vi "Setup Cursors.vi"(8 "error in (no error)":errorcluster, 11 "data":waveform(dbl)[](array[waveform])) -> (0 "error out":errorcluster, 1 "Cursor List 2":T1(array[cluster]), 2 "Cursor List":T1(array[cluster]), 3 "waveform out":waveform(dbl), 5 "duration":dbl)   [LabVIEW 2020]
uses:
  <vilib>/Waveform/WDTOps.llb/WDT Waveform Duration DBL.vi
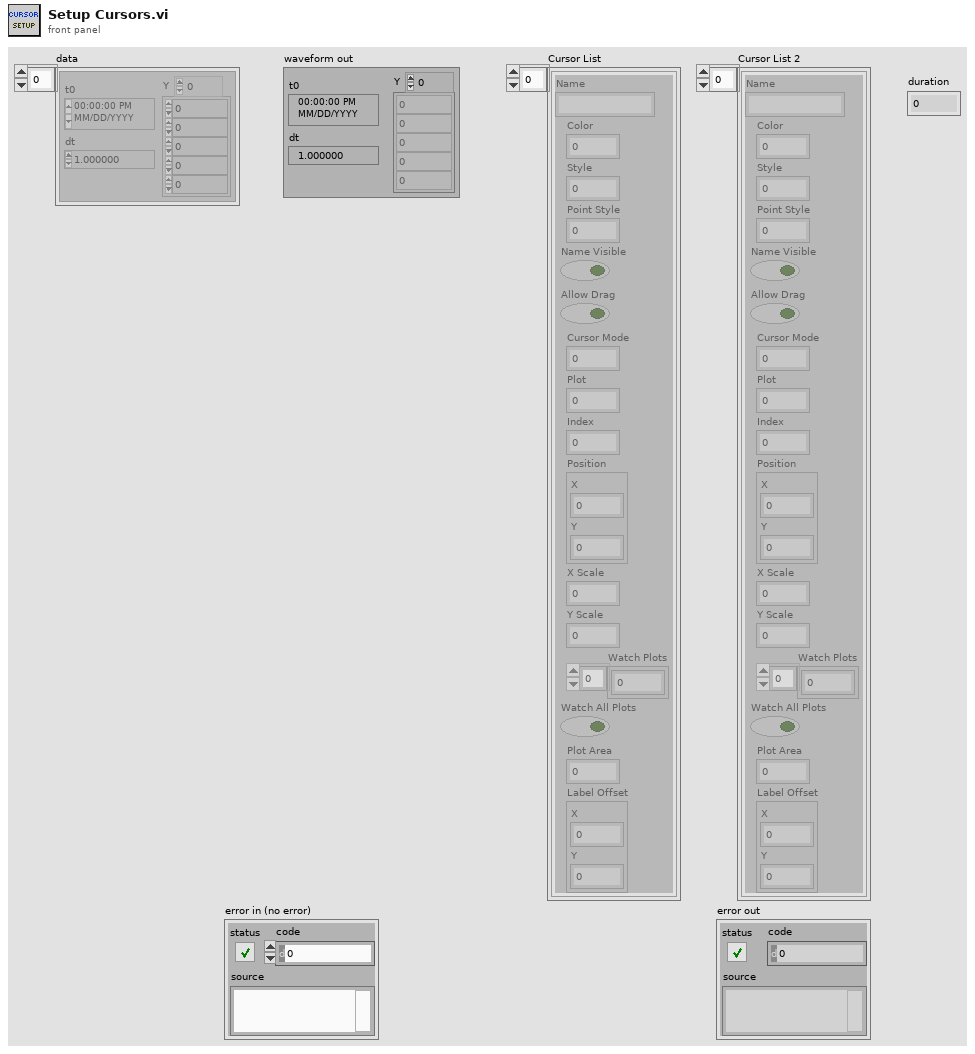
[diagram p1: front panel]
types:
  T1 = cluster{"Name":string, "Color":u32, "Style":u8, "Point Style":u8, "Name Visible":bool, "Allow Drag":bool, "Cursor Mode":u32, "Plot":i32, "Index":i32, "Position":cluster{"X":dbl, "Y":dbl}, "X Scale":u32, "Y Scale":u32, "Watch Plots":i32[], "Watch All Plots":bool, "Plot Area":i32, "Label Offset":cluster{"X":dbl, "Y":dbl}}[]
  T2 = cluster{"Name":string, "Color":u32, "Style":u8, "Point Style":u8, "Name Visible":bool, "Allow Drag":bool, "Cursor Mode":u32, "Plot":i32, "Index":i32, "Position":cluster{"X":dbl, "Y":dbl}, "X Scale":u32, "Y Scale":u32, "Watch Plots":i32[], "Watch All Plots":bool, "Plot Area":i32, "Label Offset":cluster{"X":dbl, "Y":dbl}}
  T3 = cluster{"Cursor List[0]":cluster{"Name":string, "Color":u32, "Style":u8, "Point Style":u8, "Name Visible":bool, "Allow Drag":bool, "Cursor Mode":u32, "Plot":i32, "Index":i32, "Position":cluster{"X":dbl, "Y":dbl}, "X Scale":u32, "Y Scale":u32, "Watch Plots":i32[], "Watch All Plots":bool, "Plot Area":i32, "Label Offset":cluster{"X":dbl, "Y":dbl}}, "Cursor List[1]":cluster{"Name":string, "Color":u32, "Style":u8, "Point Style":u8, "Name Visible":bool, "Allow Drag":bool, "Cursor Mode":u32, "Plot":i32, "Index":i32, "Position":cluster{"X":dbl, "Y":dbl}, "X Scale":u32, "Y Scale":u32, "Watch Plots":i32[], "Watch All Plots":bool, "Plot Area":i32, "Label Offset":cluster{"X":dbl, "Y":dbl}}, "Cursor List[2]":cluster{"Name":string, "Color":u32, "Style":u8, "Point Style":u8, "Name Visible":bool, "Allow Drag":bool, "Cursor Mode":u32, "Plot":i32, "Index":i32, "Position":cluster{"X":dbl, "Y":dbl}, "X Scale":u32, "Y Scale":u32, "Watch Plots":i32[], "Watch All Plots":bool, "Plot Area":i32, "Label Offset":cluster{"X":dbl, "Y":dbl}}, "Cursor List[3]":cluster{"Name":string, "Color":u32, "Style":u8, "Point Style":u8, "Name Visible":bool, "Allow Drag":bool, "Cursor Mode":u32, "Plot":i32, "Index":i32, "Position":cluster{"X":dbl, "Y":dbl}, "X Scale":u32, "Y Scale":u32, "Watch Plots":i32[], "Watch All Plots":bool, "Plot Area":i32, "Label Offset":cluster{"X":dbl, "Y":dbl}}, "Cursor List[4]":cluster{"Name":string, "Color":u32, "Style":u8, "Point Style":u8, "Name Visible":bool, "Allow Drag":bool, "Cursor Mode":u32, "Plot":i32, "Index":i32, "Position":cluster{"X":dbl, "Y":dbl}, "X Scale":u32, "Y Scale":u32, "Watch Plots":i32[], "Watch All Plots":bool, "Plot Area":i32, "Label Offset":cluster{"X":dbl, "Y":dbl}}, "Cursor List[5]":cluster{"Name":string, "Color":u32, "Style":u8, "Point Style":u8, "Name Visible":bool, "Allow Drag":bool, "Cursor Mode":u32, "Plot":i32, "Index":i32, "Position":cluster{"X":dbl, "Y":dbl}, "X Scale":u32, "Y Scale":u32, "Watch Plots":i32[], "Watch All Plots":bool, "Plot Area":i32, "Label Offset":cluster{"X":dbl, "Y":dbl}}, "Cursor List[6]":cluster{"Name":string, "Color":u32, "Style":u8, "Point Style":u8, "Name Visible":bool, "Allow Drag":bool, "Cursor Mode":u32, "Plot":i32, "Index":i32, "Position":cluster{"X":dbl, "Y":dbl}, "X Scale":u32, "Y Scale":u32, "Watch Plots":i32[], "Watch All Plots":bool, "Plot Area":i32, "Label Offset":cluster{"X":dbl, "Y":dbl}}, "Cursor List[7]":cluster{"Name":string, "Color":u32, "Style":u8, "Point Style":u8, "Name Visible":bool, "Allow Drag":bool, "Cursor Mode":u32, "Plot":i32, "Index":i32, "Position":cluster{"X":dbl, "Y":dbl}, "X Scale":u32, "Y Scale":u32, "Watch Plots":i32[], "Watch All Plots":bool, "Plot Area":i32, "Label Offset":cluster{"X":dbl, "Y":dbl}}, "Cursor List[8]":cluster{"Name":string, "Color":u32, "Style":u8, "Point Style":u8, "Name Visible":bool, "Allow Drag":bool, "Cursor Mode":u32, "Plot":i32, "Index":i32, "Position":cluster{"X":dbl, "Y":dbl}, "X Scale":u32, "Y Scale":u32, "Watch Plots":i32[], "Watch All Plots":bool, "Plot Area":i32, "Label Offset":cluster{"X":dbl, "Y":dbl}}}
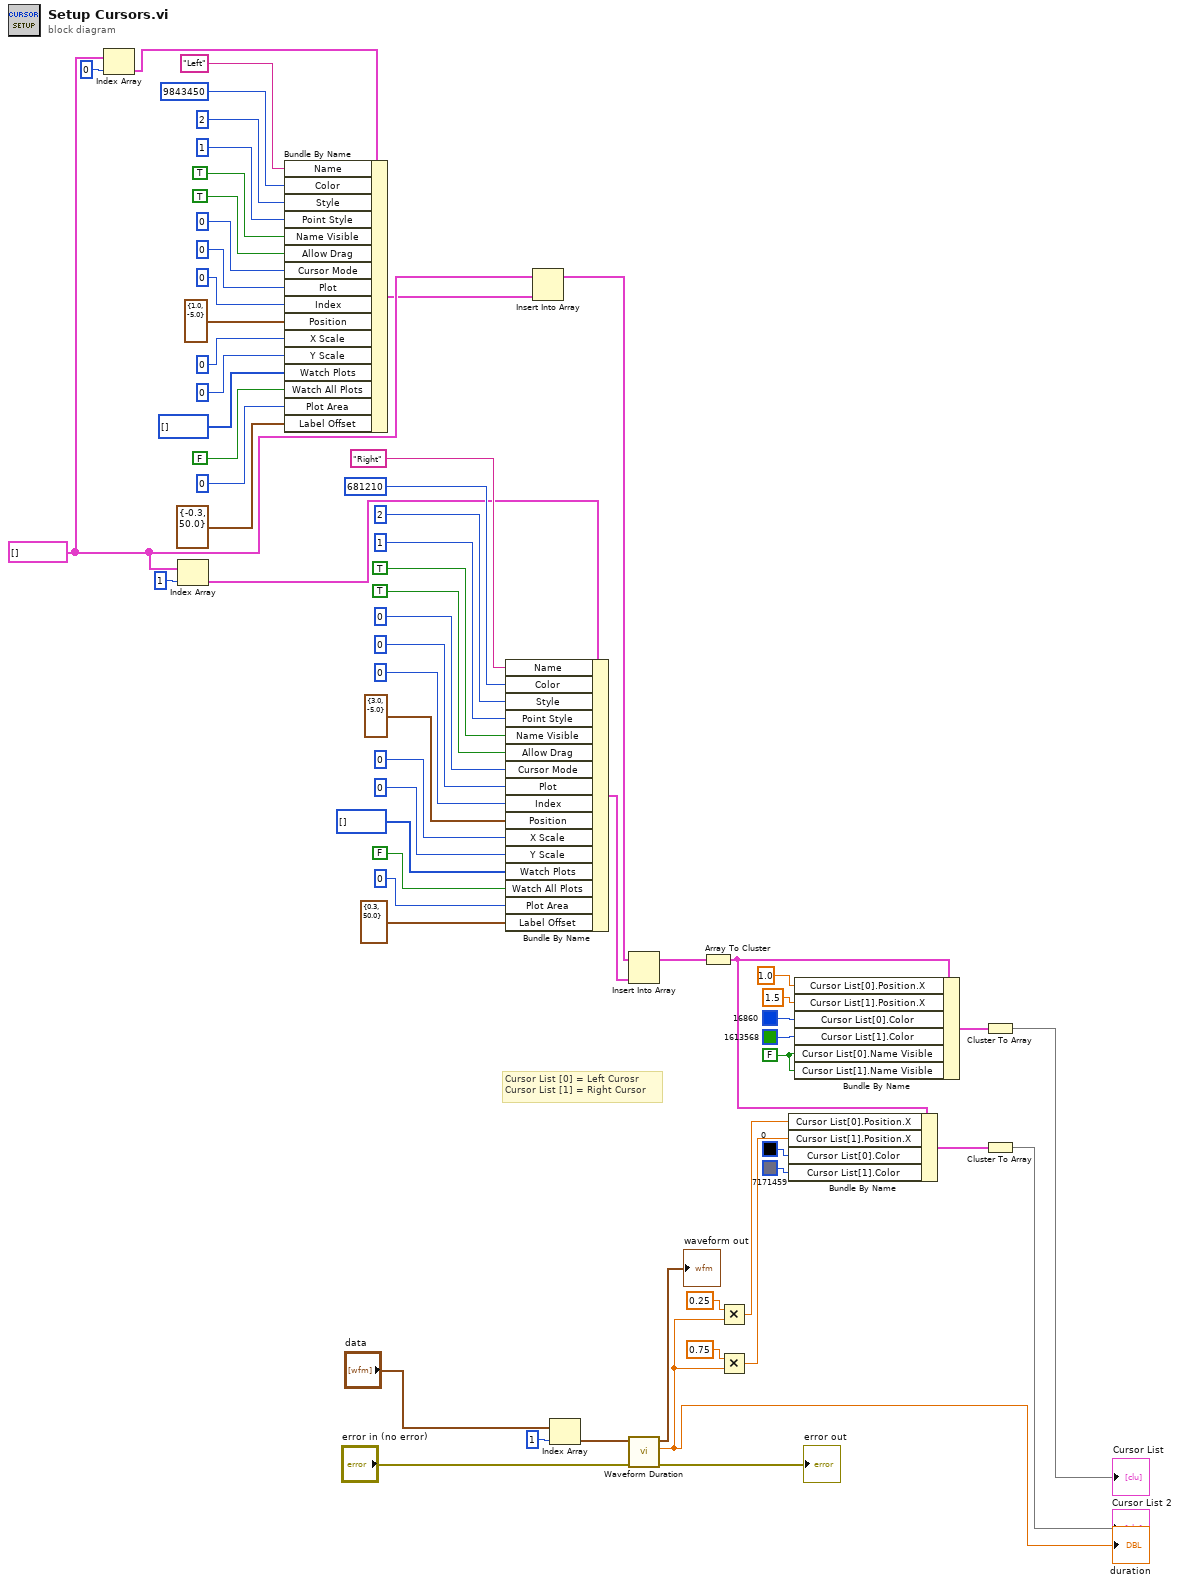
[diagram p0: block diagram]
diagram:
  w57 = T1 [] ("Cursor List")
  w11 = FALSE ("Cursor List[1].Name Visible")
  # "Cursor List [0] = Left Curosr\nCursor List [1] = Right Cursor"
  n1 = Index Array(array=w57, index=0) -> (element=w20:T2)
  n2 = Index Array(array=w57, index=1) -> (element=w24:T2)
  n3 = Bundle By Name(cluster=w20, "Name"="Left", "Color"=u32 9843450, "Style"=u8 2, "Point Style"=u8 1, "Name Visible"=TRUE, "Allow Drag"=TRUE, "Cursor Mode"=u32 0, "Plot"=0, "Index"=0, "Position"=cluster{"X":dbl, "Y":dbl} {"X"=1.0, "Y"=-5.0}, "X Scale"=u32 0, "Y Scale"=u32 0, "Watch Plots"=i32[] [], "Watch All Plots"=FALSE, "Plot Area"=0, "Label Offset"=cluster{"X":dbl, "Y":dbl} {"X"=-0.3, "Y"=50.0}) -> (w22:T2)
  n4 = Bundle By Name(cluster=w24, "Name"="Right", "Color"=u32 681210, "Style"=u8 2, "Point Style"=u8 1, "Name Visible"=TRUE, "Allow Drag"=TRUE, "Cursor Mode"=u32 0, "Plot"=0, "Index"=0, "Position"=cluster{"X":dbl, "Y":dbl} {"X"=3.0, "Y"=-5.0}, "X Scale"=u32 0, "Y Scale"=u32 0, "Watch Plots"=i32[] [], "Watch All Plots"=FALSE, "Plot Area"=0, "Label Offset"=cluster{"X":dbl, "Y":dbl} {"X"=0.3, "Y"=50.0}) -> (w23:T2)
  n5 = Insert Into Array(array=w57, new element=w22) -> (w21:T1)  [unwired: 1 in]
  n6 = Index Array(array="data", index=1) -> (element=w59:waveform(dbl))
  n7 = Insert Into Array(array=w21, new element=w23) -> (w58:T1)  [unwired: 1 in]
  n8 = call-poly <vilib>:"Waveform Duration.vi"("error in (no error)"="error in (no error)", "waveform in"=w59) -> ("error out"=→"error out":errorcluster, "duration"=w64:dbl, "waveform out"=→"waveform out":waveform(dbl))  [unwired: 7 in]
  "duration" <- w64
  n9 = Array To Cluster(array=w58) -> (cluster=w6:T3)
  n10 = Multiply(x=0.25 ("Cursor List[0].Position.X"), y=w64) -> (x*y=w16:dbl)
  n11 = Multiply(x=0.75 ("Cursor List[1].Position.X"), y=w64) -> (x*y=w17:dbl)
  n12 = Bundle By Name(cluster=w6, "Cursor List[0].Position.X"=w16, "Cursor List[1].Position.X"=w17, "Cursor List[0].Color"=u32 0, "Cursor List[1].Color"=u32 7171459) -> (w2:T3)
  n13 = Bundle By Name(cluster=w6, "Cursor List[0].Position.X"=1.0, "Cursor List[1].Position.X"=1.5 ("Cursor List[0].Position.Y"), "Cursor List[0].Color"=u32 16860, "Cursor List[1].Color"=u32 1613568, "Cursor List[0].Name Visible"=w11, "Cursor List[1].Name Visible"=w11) -> (w3:T3)
  n14 = Cluster To Array(cluster=w3) -> (array=→"Cursor List":T1)
  n15 = Cluster To Array(cluster=w2) -> (array=→"Cursor List 2":T1)
